vi "set_source_parameter.vi"(6 "Parameter":variant, 8 "error in (no error)":errorcluster, 9 "Source number":u8=1 min=1 max=50 step=1, 10 "Source parameter":T1 items=["DAC Output", "Shutter Output", "Number of Crucibles", "Crucible Output", "Turret Feedback", "Turret Input", "Turret Delay (s)"], 11 "VISA resource name":refnum<visa-resource-name>) -> (0 "error out":errorcluster, 3 "VISA resource name out":refnum<visa-resource-name>)   [LabVIEW 2018]
doc: "Set the density of a material."
uses:
  Low Level/source_parameter_ring.ctl
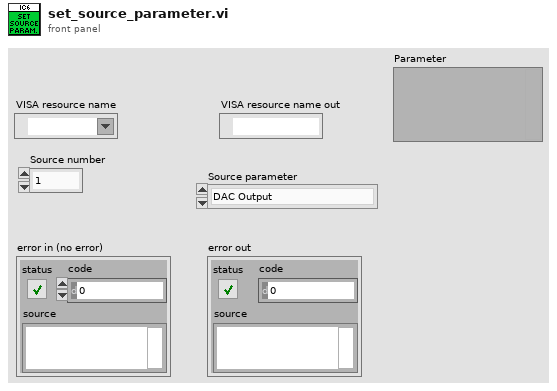
[diagram p1: front panel]
types:
  T1 = typedef "source_parameter_ring.ctl" = u16
  T2 = enum16{"Source", "General", "Input name", "Process name", "Logic", "Material", "Material name", "Output name", "Process", "Sensor", "Output type", "User message", "Layer", ""}
  T3 = enum16{"Hello", "Query", "Remote action", "Status", "Update"}
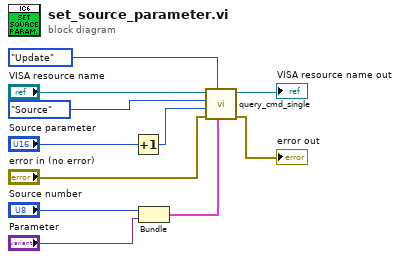
[diagram p0: block diagram]
diagram:
  n1 = Increment(x="Source parameter") -> (x+1=w4:T1)
  n2 = Bundle("Source number"="Source number", "Parameter"="Parameter") -> (w2:cluster{"Source number":u8, "Parameter":variant})  [unwired: 1 in]
  n3 = call "query_cmd_single.vi"("Parameter"=w2, "Command group"=T3."Update", "error in (no error)"="error in (no error)", "Command ID"=w4, "Command subgroup"=T2."Source", "VISA resource name"="VISA resource name") -> ("error out"=→"error out":errorcluster, "VISA resource name out"=→"VISA resource name out":refnum<visa-resource-name>)  [unwired: 1 in, 3 out]
